vi "Read Laser Type .vi"(8 "error in (no error)":errorcluster, 11 "Laser in":refnum<class "Laser.lvclass">) -> (0 "error out":errorcluster, 2 "Laser Type":T1, 3 "Laser out":refnum<class "Laser.lvclass">)   [LabVIEW 2018, in "Laser.lvlib" / "Laser.lvclass"]
uses:
  Laser.lvclass
  Custom Controls/Laser Type.ctl
  Laser.lvclass/Laser.ctl
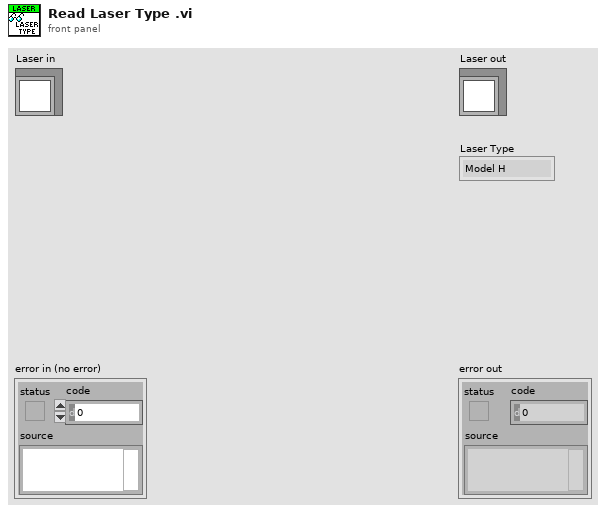
[diagram p1: front panel]
types:
  T1 = typedef "Laser.lvlib/Laser.lvclass/Laser Type.ctl" = enum16{"Model H", "Model I"}
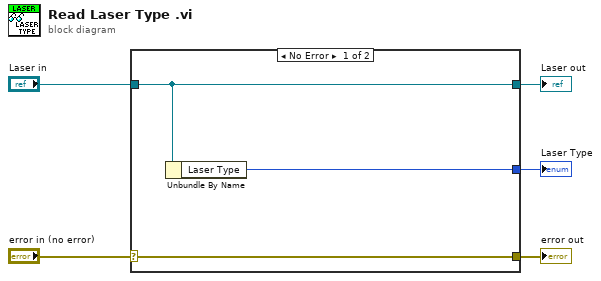
[diagram p0: block diagram]
diagram:
  n1 = case shown="No Error" "error in (no error)" {
    selector: "error in (no error)" -> [w8 w9]
    tunnel: [w8 w9] -> w4
    tunnel: [w7 w10] -> w2
    tunnel: "Laser in" -> [w7 w10]
    tunnel: [w6 _] -> w1
    frame No Error {
      n2 = Unbundle By Name(w7) -> ("Laser Type"=w6:T1)
    }
    frame Error {
    }
  }
  "error out" <- w4
  "Laser out" <- w2
  "Laser Type" <- w1
